vi "disable.vi"(8 "error in (no error)":errorcluster, 11 "DL090603DAQmxOnOffEmissionSensor in":refnum<class "DetectorDL090603DAQmxOnOff.lvclass">=refnum) -> (0 "error out":errorcluster, 3 "DL090603DAQmxOnOffEmissionSensor out":refnum<class "DetectorDL090603DAQmxOnOff.lvclass">)   [LabVIEW 2010, in "DetectorDL090603DAQmxOnOff.lvclass"]
uses:
  DetectorDL090603DAQmxOnOff.lvclass
  DetectorDL090603DAQmxOnOff.lvclass/DetectorDL090603DAQmxOnOff.ctl
  DigitalOut/DigitalOutDL110325DAQmx/DigitalOutDL110325DAQmx/DigitalOutDL110325DAQmx.lvclass
  GenericDetector/GenericDetector/GenericDetector.lvclass
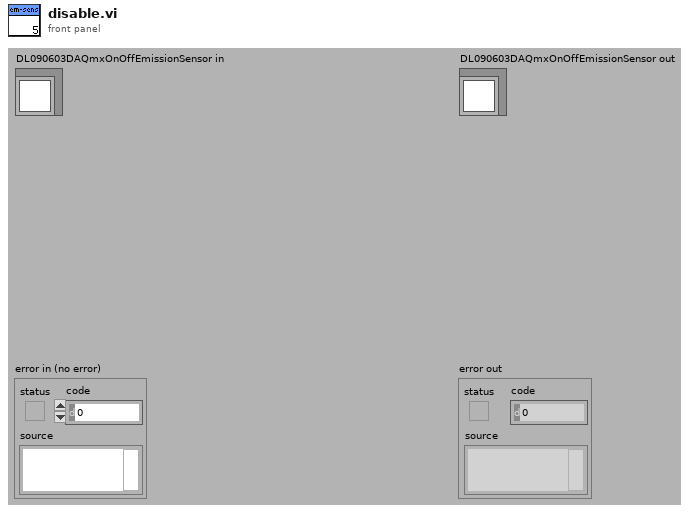
[diagram p1: front panel]
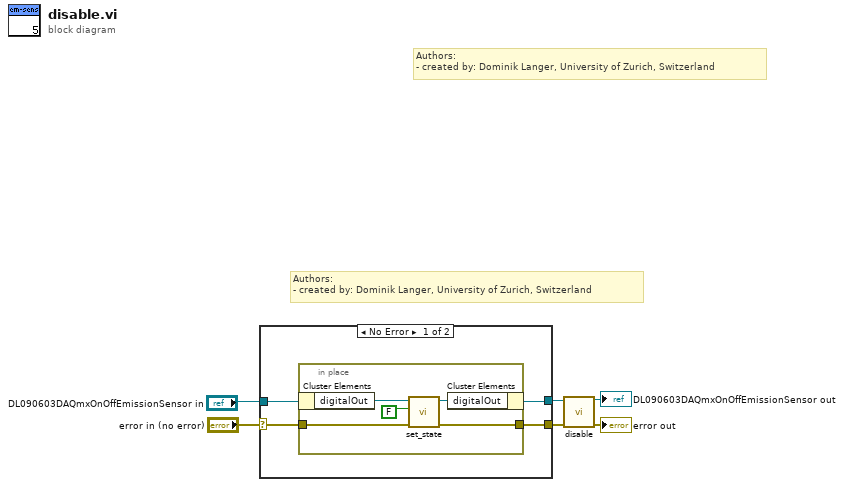
[diagram p0: block diagram]
diagram:
  # "Authors: \n- created by: Dominik Langer, University of Zurich, Switzerland"
  # "Authors: \n- created by: Dominik Langer, University of Zurich, Switzerland"
  n1 = case shown="No Error" "error in (no error)" {
    selector: "error in (no error)" -> [w10 w17]
    tunnel: [w9 w17] -> w2
    tunnel: [w7 w16] -> w4
    tunnel: "DL090603DAQmxOnOffEmissionSensor in" -> [w8 w16]
    frame No Error {
      n2 = in-place {
        in-place-border: w10 -> [w15]
        in-place-border: [w14] -> w9
        n3 = in-place-cluster #1(w8) -> ("digitalOut"=w12:refnum<class "DigitalOutDL110325DAQmx.lvclass">)
        n4 = call-dynamic "set_state.vi"("error in (no error)"=w15, "state"=FALSE ("data"), "DAQmxDigitalOut in"=w12) -> ("error out"=w14:errorcluster, "DAQmxDigitalOut out"=w11:refnum<class "DigitalOutDL110325DAQmx.lvclass">)  [unwired: 7 in]
        n5 = in-place-cluster #1("digitalOut"=w11) -> (w7:refnum<class "DetectorDL090603DAQmxOnOff.lvclass">)
      }
    }
    frame Error {
    }
  }
  n6 = call-parent "disable.vi"("error in (no error)"=w2, "GenericEmissionSensor in"=w4) -> ("error out"=→"error out":errorcluster, "GenericEmissionSensor out"=→"DL090603DAQmxOnOffEmissionSensor out":refnum<class "DetectorDL090603DAQmxOnOff.lvclass">)  [unwired: 8 out]
